vi "Normalize with Lowest Den Term.vi"   [LabVIEW 2014, in "NI_AALPro.lvlib"]
doc: "Normalizes numerator and denominator polynomials with the lowest denominator term. The data types you wire to the <B>Numerator</B> and <B>Denominator</B> inputs determine the polymorphic instance to use."
uses:
  NI_AALPro.lvlib
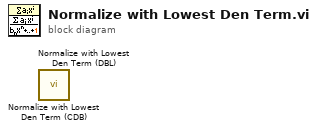
[diagram p0: block diagram]
diagram:
  n1 = call "Normalize with Lowest Den Term (CDB).vi"() -> ()  [unwired: 9 in, 3 out]
  n2 = call "Normalize with Lowest Den Term (DBL).vi"() -> ()  [unwired: 9 in, 3 out]
